vi "CRYGet Formula & Result Variable.vi"(11 "String":string) -> (1 "Formula Out":string[](array[string]), 2 "Result Variable":string[](array[string]), 3 "Out string":string)   [LabVIEW 2013]
uses:
  <vilib>/Utility/error.llb/whitespace.ctl
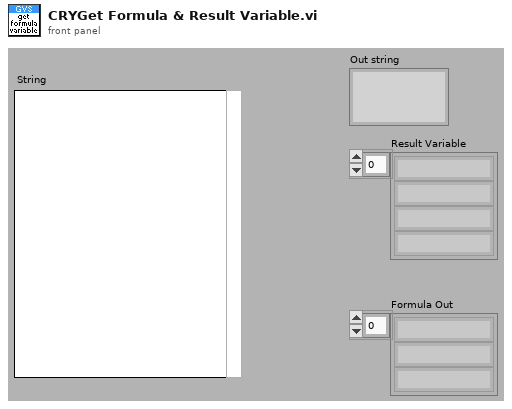
[diagram p1: front panel]
types:
  T1 = typedef "whitespace.ctl" = u16
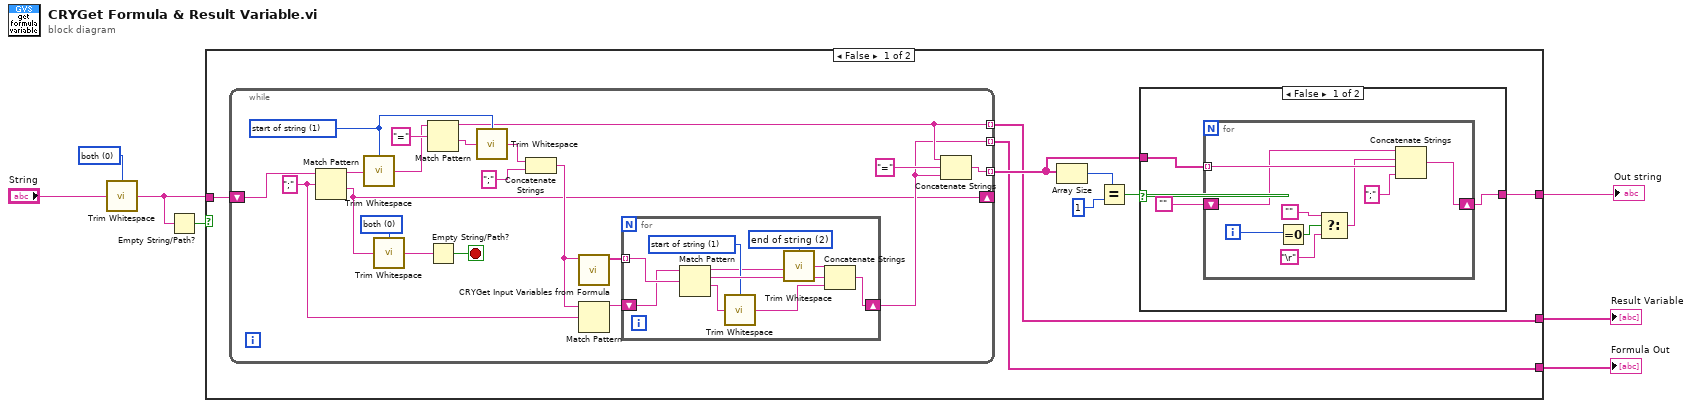
[diagram p0: block diagram]
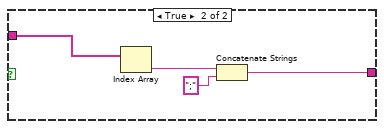
[diagram p2: hidden frame]
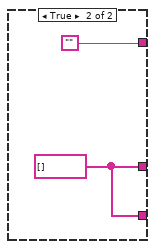
[diagram p3: hidden frame]
diagram:
  w1 = T1 0 items=["both", "start of string", "end of string"] ("location (both)")
  n1 = call <vilib>:"Trim Whitespace.vi"("string"="String", "location (both)"=w1) -> ("trimmed string"=w2:string)
  n2 = Empty String/Path?(string/path=w2) -> (empty?=w4:bool)
  n3 = case shown="False" w4 {
    tunnel: w2 -> [w11 _]
    tunnel: [w10 ""] -> w7
    tunnel: [w9 w62] -> w6
    tunnel: [w8 w62] -> w5
    frame False {
      n4 = while {
        tunnel: [w20] -> w12 mode=indexing
        shift-right: [w18] -> _
        shift-left: w11 -> [w35]
        tunnel: [w23] -> w9 mode=indexing
        tunnel: [w21] -> w8 mode=indexing
        stop <- w19 stop-if-true
        w16 = T1 0 items=["both", "start of string", "end of string"] ("location (both)")
        w30 = T1 1 items=["both", "start of string", "end of string"] ("location (both)")
        w25 = ";" ("regular expression")
        n5 = Match Pattern(string=w35, regular expression=w25) -> (before substring=w34:string, after substring=w18:string)  [unwired: 1 in, 2 out]
        n6 = call <vilib>:"Trim Whitespace.vi"("string"=w34, "location (both)"=w30) -> ("trimmed string"=w32:string)
        n7 = call <vilib>:"Trim Whitespace.vi"("string"=w18, "location (both)"=w16) -> ("trimmed string"=w17:string)
        n8 = Match Pattern(string=w32, regular expression="=") -> (before substring=w23:string, after substring=w31:string)  [unwired: 1 in, 2 out]
        n9 = Empty String/Path?(string/path=w17) -> (empty?=w19:bool)
        n10 = call <vilib>:"Trim Whitespace.vi"("string"=w31, "location (both)"=w30) -> ("trimmed string"=w29:string)
        n11 = Concatenate Strings(w29, ";" ("string")) -> (w26:string)
        n12 = call "CRYGet Input Variables from Formula.vi"("Formula string"=w26) -> ("Variables Out"=w27:string[])  [unwired: 10 in]
        n13 = Match Pattern(string=w26, regular expression=w25) -> (before substring=w24:string)  [unwired: 1 in, 3 out]
        n14 = for {
          tunnel: w27 -> [w45] mode=indexing
          shift-right: [w40] -> w21
          shift-left: w24 -> [w39]
          w36 = T1 2 items=["both", "start of string", "end of string"] ("location (both)")
          w42 = T1 1 items=["both", "start of string", "end of string"] ("location (both)")
          n15 = Match Pattern(string=w39, regular expression=w45) -> (before substring=w37:string, match substring=w44:string, after substring=w43:string)  [unwired: 1 in, 1 out]
          n16 = call <vilib>:"Trim Whitespace.vi"("string"=w43, "location (both)"=w42) -> ("trimmed string"=w41:string)
          n17 = call <vilib>:"Trim Whitespace.vi"("string"=w37, "location (both)"=w36) -> ("trimmed string"=w38:string)
          n18 = Concatenate Strings(w38, w44, w41) -> (w40:string)
        }
        n19 = Concatenate Strings(w23, "=" ("string"), w21) -> (w20:string)
      }
      n20 = Array Size(array=w12) -> (size(s)=w13:i32)
      n21 = Equal?(x=w13, y=1) -> (x = y?=w14:bool)
      n22 = case shown="False" w14 {
        tunnel: w12 -> [w48 w61]
        tunnel: [w47 w58] -> w10
        frame False {
          n23 = for {
            tunnel: w48 -> [w57] mode=indexing
            shift-right: [w56] -> w47
            shift-left: "" -> [w52]
            i -> [w51]
            n24 = Equal To 0?(x=w51) -> (x = 0?=w55:bool)
            n25 = Select(t="", s=w55, f="\r") -> (s? t:f=w53:string)
            n26 = Concatenate Strings(w52, w53, w57, ";" ("string")) -> (w56:string)
          }
        }
        frame True {
          n27 = Index Array(array=w61) -> (element=w60:string)  [unwired: 1 in]
          n28 = Concatenate Strings(w60, ";" ("string")) -> (w58:string)
        }
      }
    }
    frame True {
      w62 = string[] []
    }
  }
  "Formula Out" <- w5
  "Result Variable" <- w6
  "Out string" <- w7
